vi "Create.vi"(10 "Role":T1, 11 "Username":string) -> (3 "User":refnum<class "User.lvclass">)   [LabVIEW 2026, in "User.lvclass"]
uses:
  User.lvclass
  User.lvclass/User.ctl
  Typedefs/enums/Role Enum.ctl
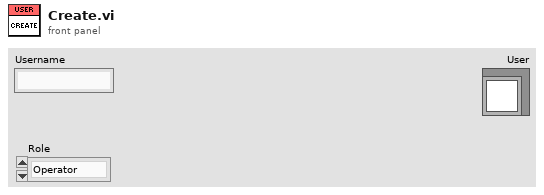
[diagram p1: front panel]
types:
  T1 = typedef "Role Enum.ctl" = enum16{"Operator", "Engineer", "Admin"}
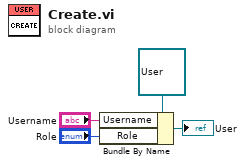
[diagram p0: block diagram]
diagram:
  n1 = Bundle By Name(cluster=refnum<class "User.lvclass"> refnum ("User.lvclass"), "Username"="Username", "Role"="Role") -> (→"User":refnum<class "User.lvclass">)
